vi "SEARCH-FOR-TAG.vi"(9 "tag":string, 11 "tbl.list":T1[](array[typedef]) {"tMsgData"."dwID" format="%03x"; "last.frame"."payload" format="%x"; "last.frame"."timestamp" format="%<%.7X\n%x>T"; "last.frame"."type" items=["CAN Data"=0, "CAN Remote"=1, "CAN Bus Error"=2, "J1939 Data"=192, "Delay"=224, "Log Trigger"=225, "Start Trigger"=226]; "last.frame"."identifier" format="%x"}) -> (1 "idx":i32, 3 "tbl.list out":T1[](array[typedef]) {"tMsgData"."dwID" format="%03x"; "last.frame"."payload" format="%x"; "last.frame"."timestamp" format="%<%.7X\n%x>T"; "last.frame"."type" items=["CAN Data"=0, "CAN Remote"=1, "CAN Bus Error"=2, "J1939 Data"=192, "Delay"=224, "Log Trigger"=225, "Start Trigger"=226]; "last.frame"."identifier" format="%x"})   [LabVIEW 2015, in "bAPPdata.lvclass"]
uses:
  bAPPdata.lvclass
  table-contents.ctl
  subs/frame.type.ctl
  <vilib>/xnet/xnet.llb/XNET Frame CAN.ctl
  <vilib>/xnet/xnet.llb/XNET Frame Type CAN.ctl
  nMsgData.ctl
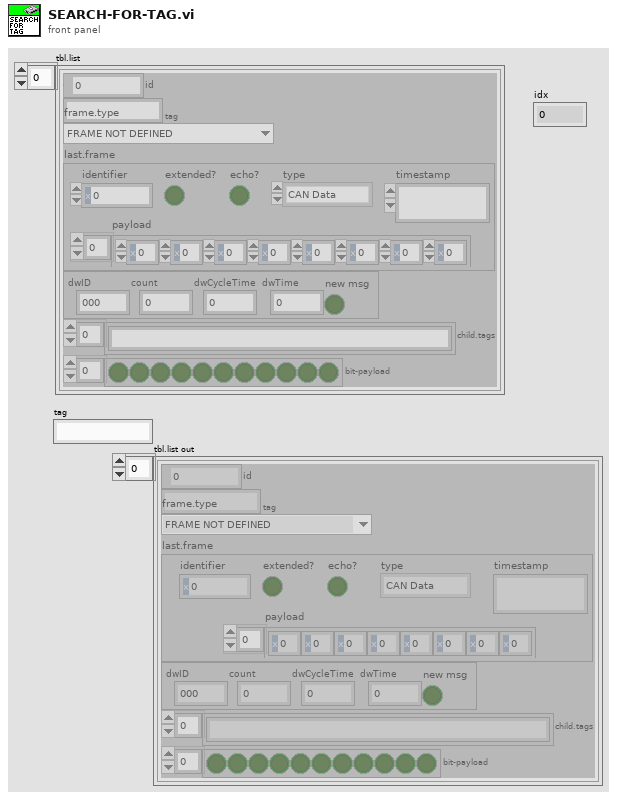
[diagram p1: front panel]
types:
  T1 = typedef "bAPPdata.lvclass/table-contents.ctl" = cluster{"id":u32, "tag":string, "frame.type":T2, "last.frame":T3, "tMsgData":T5, "child.tags":string[], "bit-payload":bool[]}
  T2 = typedef "frame.type.ctl" = enum16{"FRAME NOT DEFINED", "DUT OUTPUT FRAME", "DUT INPUT FRAME"}
  T3 = typedef "XNET Frame CAN.ctl" = cluster{"timestamp":timestamp, "payload":u8[], "identifier":u32, "type":T4, "extended?":bool, "echo?":bool}
  T4 = typedef "XNET Frame Type CAN.ctl" = u8
  T5 = typedef "nMsgData.ctl" = cluster{"dwID":u32, "count":u32, "dwCycleTime":dbl, "dwTime":dbl, "new msg":bool}
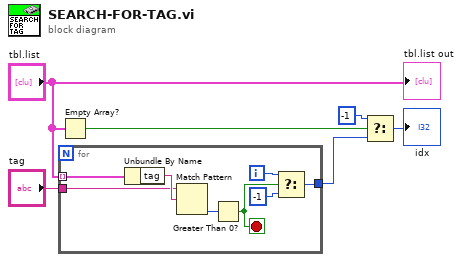
[diagram p0: block diagram]
diagram:
  n1 = for {
    tunnel: "tbl.list" -> [w14] mode=indexing
    tunnel: "tag" -> [w9]
    tunnel: [w11] -> w3
    i -> [w13]
    stop <- w7 stop-if-true
    n2 = Unbundle By Name(w14) -> ("tag"=w10:string)
    n3 = Match Pattern(string=w9, regular expression=w10) -> (offset past match=w8:i32)  [unwired: 1 in, 3 out]
    n4 = Greater Than 0?(x=w8) -> (x > 0?=w7:bool)
    n5 = Select(t=w13, s=w7, f=-1) -> (s? t:f=w11:i32)
  }
  n6 = Empty Array?(array="tbl.list") -> (empty?=w2:bool)
  n7 = Select(t=-1, s=w2, f=w3) -> (s? t:f=→"idx":i32)
  "tbl.list out" <- "tbl.list"
